vi "BypassControl.vi"(6 "Cutoff":dbl=0.15 format="%#_13g", 8 "MaxMotorChangeForward":dbl, 9 "MaxMotorChangeBackward":dbl, 10 "Current Input":dbl, 11 "Previous Input":dbl) -> (2 "In range?":bool, 3 "SetMotor":dbl)   [LabVIEW 2015]
doc: "This VI handles motor values that are changing across a deadzone.\nIf leaving a deadzone, set the output to the boundary of the deadzone (bypassing it).\nIf staying in the deadzone, set the output to 0.\nIf staying outside the deadzone, ramp the output.\nInputs:\n CurrentInput - What the current or \"previous\" motor value was\n Cutoff - The deadzone range\n DesiredInput - What the new input should be\n MaxMotorChangeForward - How quickly the motor should accelerate forwards\n MaxMotorChangeBackward - How quickly the motor should accelerate in reverse\nOutputs:\n SetMotor - The value that the motor should be set to\nCode:\n If the CurrentInput is within the cutoff AND the DesiredInput is outside the deadzone,\n then skip over the deadzone by setting the motor output to the cutoff value on the \n other side of 0\n Otherwise, enter Limited Acceleration"
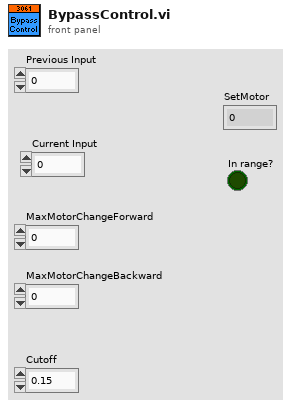
[diagram p1: front panel]
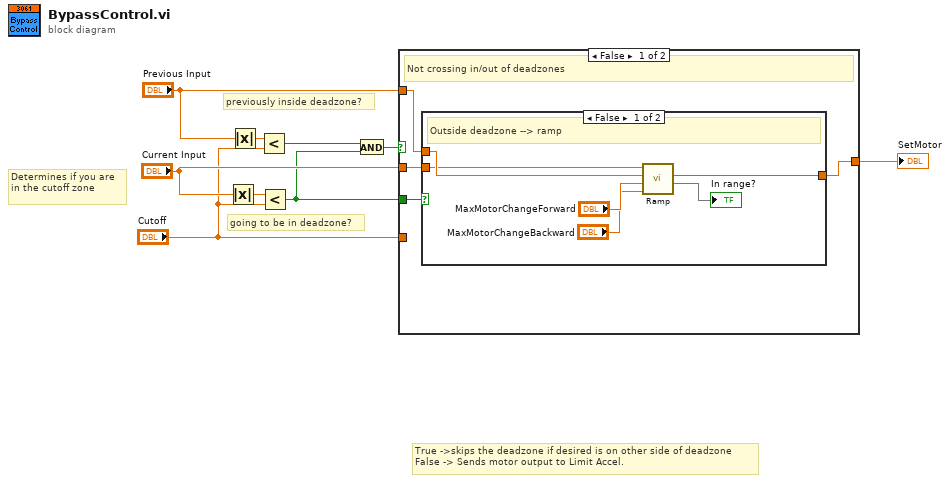
[diagram p0: block diagram]
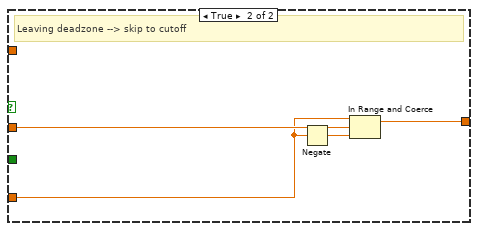
[diagram p3: hidden frame]
diagram:
  # "going to be in deadzone?"
  # "previously inside deadzone?"
  # "Determines if you are in the cutoff zone"
  # "True ->skips the deadzone if desired is on other side of deadzone\nFalse -> Sends motor output to Limit Accel."
  n1 = Absolute Value(x="Current Input") -> (abs(x)=w8:dbl)
  n2 = Absolute Value(x="Previous Input") -> (abs(x)=w9:dbl)
  n3 = Less?(x=w9, y="Cutoff") -> (x < y?=w2:bool)
  n4 = Less?(x=w8, y="Cutoff") -> (x < y?=w1:bool)
  n5 = And(x=w2, y=w1) -> (x .and. y?=w7:bool)
  n6 = case shown="False" w7 {
    tunnel: "Current Input" -> [w11 w23]
    tunnel: "Previous Input" -> [w13 _]
    tunnel: [w12 w24] -> w5
    tunnel: "Cutoff" -> [_ w21]
    tunnel: w1 -> [w10 _]
    frame False {
      # "Not crossing in/out of deadzones"
      n7 = case shown="False" w10 {
        tunnel: w13 -> [w19 _]
        tunnel: [w18 w20] -> w12
        tunnel: w11 -> [w16 w20]
        frame False {
          # "Outside deadzone --> ramp"
          n8 = call "Ramp.vi"("error in (no error)"="MaxMotorChangeBackward", 9:"MaxMotorChangeForward", "Max change (power / sec)"=w19, "Joystick in"=w16) -> (1:→"In range?", 2:w18)  [unwired: 4 in, 2 out]
        }
        frame True {
          # "Inside deadzone --> passthrough"
        }
      }
    }
    frame True {
      # "Leaving deadzone --> skip to cutoff"
      n9 = Negate(x=w21) -> (-x=w22:dbl)
      n10 = In Range and Coerce(upper limit=w21, x=w23, lower limit=w22) -> (coerced(x)=w24:dbl)  [unwired: 1 out]
    }
  }
  "SetMotor" <- w5
